vi "Basic Int trans.vi"(8 "Error In":errorcluster, 11 "int variable name":string) -> (0 "Error Out":errorcluster, 3 "resulting string":string)   [LabVIEW 2014]
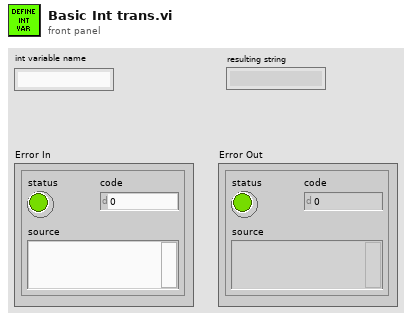
[diagram p1: front panel]
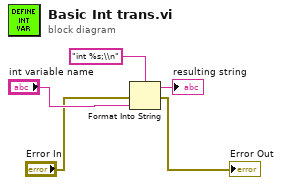
[diagram p0: block diagram]
diagram:
  n1 = Format Into String(format string="int %s;\\n", error in="Error In", "int variable name") -> (resulting string=→"resulting string":string, error out=→"Error Out":errorcluster)  [unwired: 1 in]
